vi "Weather Station UI.vi"(7 "stop":bool) -> (1 "Mise en garde":string, 2 "Historique de la température":dbl(graph))   [LabVIEW 2013]
doc: "Ceci est le VI principal du Projet Station météo. Il comporte l'interface utilisateur d'un système de mise en garde concernant la température. La température est mesurée toutes les demi-secondes ; les données sont enregistrées lorsqu'une mise en garde survient.\n\nEntrées utilisateur : Limite supérieure de température, Limite inférieure de température, Unités de température.\nSorties : Température actuelle, État de mise en garde."
uses:
  Supporting Files/Weather Station States.ctl
  Instance           1 26Saved   Weather Station UI .vi
panel:
  in  "Limite inférieure":dbl=10.0 min=0.0 max=50.0
  in  "Limite supérieure":dbl=30.0 min=0.0 max=50.0
  # "Gamme de température (C)"
  # "Canicule"
  # "Gel"
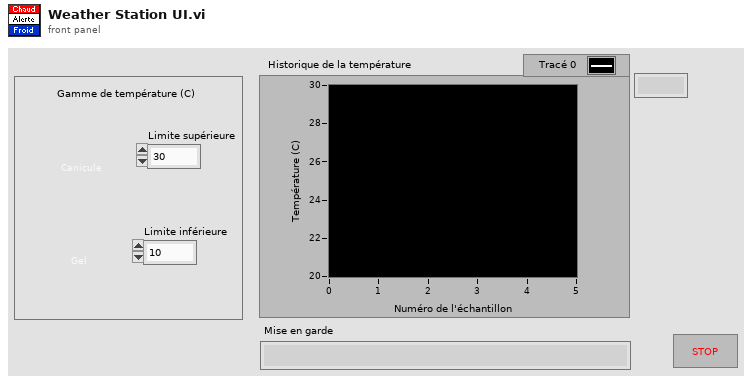
[diagram p1: front panel]
types:
  T1 = enum16{"open", "replace", "create", "open or create", "replace or create", "replace or create with confirmation"}
  T2 = typedef "Weather Station States.ctl" = enum16{"Acquisition", "Verification de la gamme", "Analyse", "Enregistrement des données", "Vérification du temps écoulé"}
  T3 = cluster{"Température":dbl, "Limite supérieure de T":dbl, "Limite inférieure de T":dbl, "Mise en garde":string}
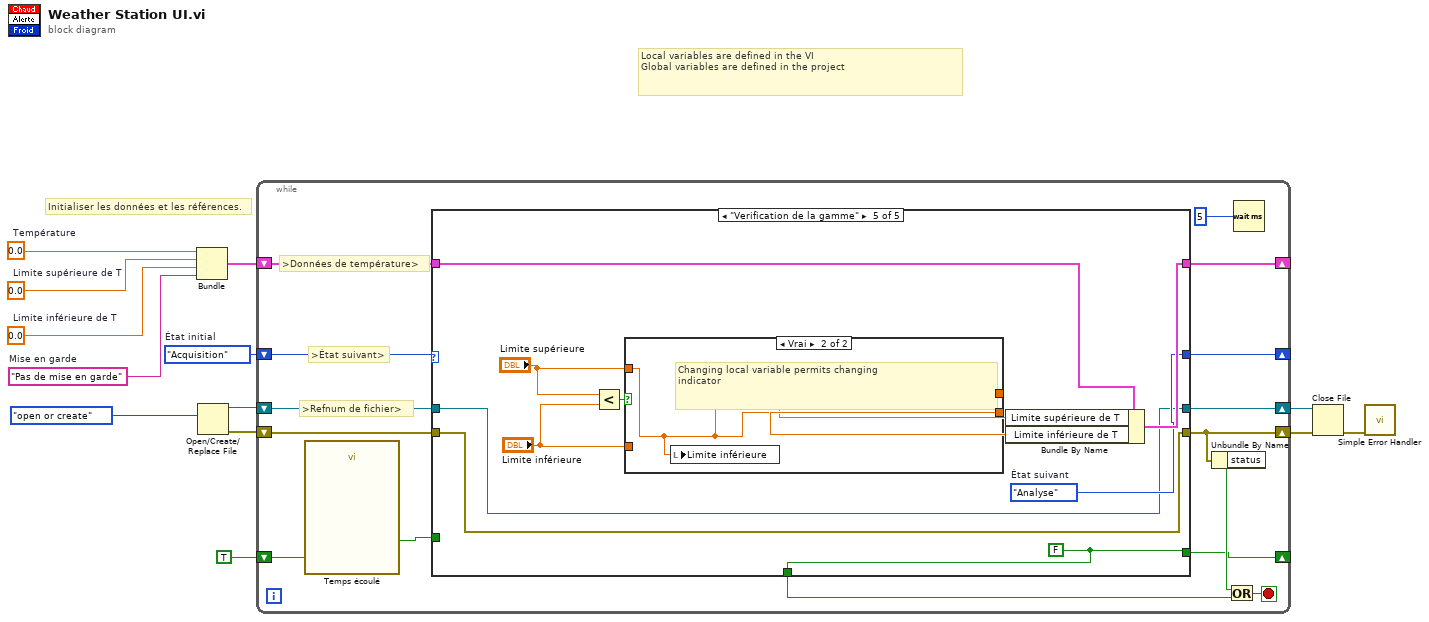
[diagram p0: block diagram]
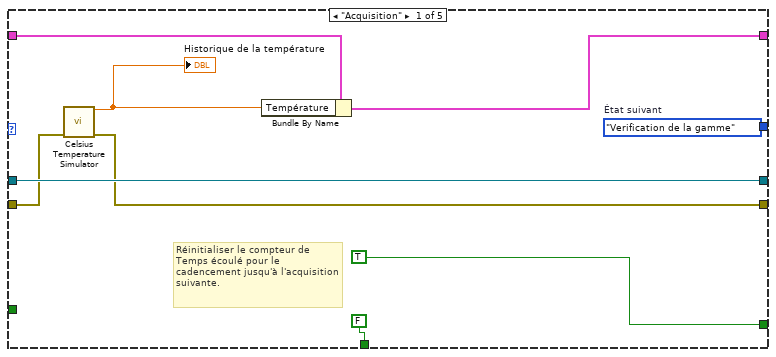
[diagram p2: hidden frame]
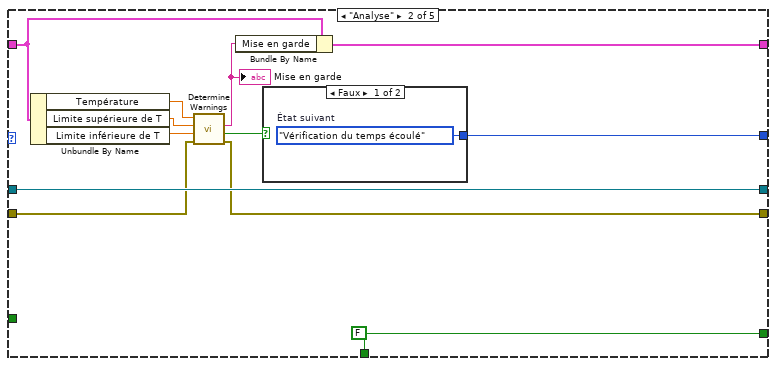
[diagram p3: hidden frame]
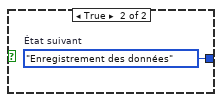
[diagram p4: hidden frame]
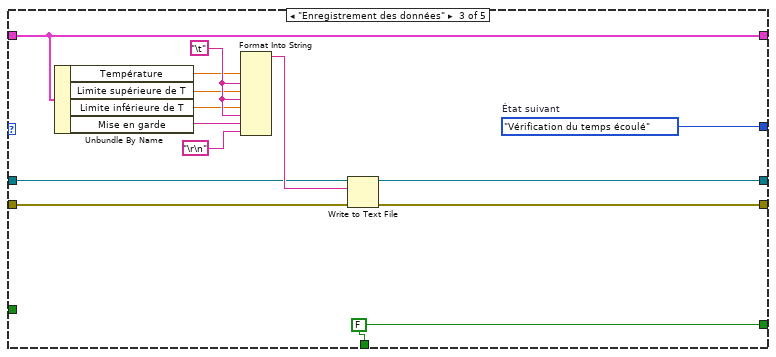
[diagram p5: hidden frame]
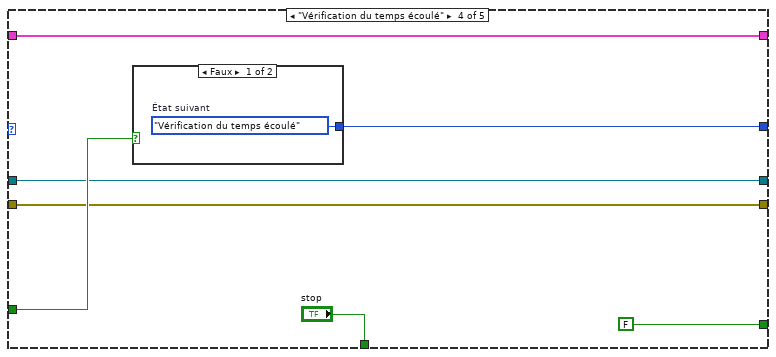
[diagram p6: hidden frame]
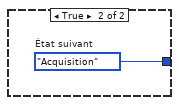
[diagram p7: hidden frame]
diagram:
  w7 = 0.0  # Limite inférieure de T
  w6 = 0.0  # Limite supérieure de T
  w8 = "Pas de mise en garde"  # Mise en garde
  w4 = 0.0  # Température
  w13 = Weather_Station_States."Acquisition"  # État initial
  # "Local variables are defined in the VI\nGlobal variables are defined in the project"
  # "Initialiser les données et les références."
  n1 = Bundle ("Assembler")("Température"=w4, "Limite supérieure de T"=w6, "Limite inférieure de T"=w7, "Mise en garde"=w8) -> (w1:T3)  [unwired: 1 out]
  n2 = Open/Create/Replace File ("Ouvrir/Créer/Remplacer un fichier")(operation (0:open)=T1."open or create") -> (refnum out=w3:refnum<file>, error out=w2:errorcluster)  [unwired: 1 in, 5 out]
  n3 = while "Boucle While" {
    shift-right: [w27] -> _
    shift-left: w13 -> [w28]
    shift-right: [w14] -> w12
    shift-left: w2 -> [w26]
    shift-right: [w15] -> _
    shift-left: w1 -> [w22]
    shift-right: [w23] -> w11
    shift-left: w3 -> [w21]
    shift-right: [w16] -> _
    shift-left: TRUE ("stop") -> [w18]
    stop <- w25 stop-if-true
    # ">Données de température>"
    # ">Refnum de fichier>"
    # ">État suivant>"
    n4 = call "Temps écoulé"("Reset"=w18) -> ("Time has Elapsed"=w17:bool)  [unwired: 4 in, 14 out]
    n5 = case "Structure Condition" shown="\"Verification de la gamme\"" w28 {
      tunnel: [w37 w47 w65 w71 w78] -> w27
      tunnel: [w29 w40 w63 w67 w77] -> w14
      tunnel: w26 -> [w30 w41 w64 w67 w77]
      tunnel: [w36 w49 w62 w68 w75] -> w23
      tunnel: [w32 w42 w52 w66 w79] -> w15
      tunnel: w22 -> [w33 w43 w52 w66 w82]
      tunnel: w21 -> [w36 w49 w60 w68 w75]
      tunnel: [FALSE ("stop") w48 w58 "stop" w76] -> w20
      tunnel: w17 -> [_ _ _ w72 _]
      tunnel: [TRUE ("stop") w48 w58 FALSE ("stop") w76] -> w16
      frame "Acquisition" {
        w37 = Weather_Station_States."Verification de la gamme"  # État suivant
        # "Réinitialiser le compteur de Temps écoulé pour le cadencement jusqu'à l'acquisition suivante."
        n6 = call "Celsius Temperature Simulator.vi"("entrée d'erreur (pas d'erreur)"=w30) -> ("Température"=w31:dbl, "sortie d'erreur"=w29:errorcluster)  [unwired: 13 out]
        "Historique de la température" <- w31
        n7 = Bundle By Name(cluster=w33, "Température"=w31) -> (w32:T3)
      }
      frame "Analyse" {
        w48 = FALSE ("stop")
        n8 = Unbundle By Name(w43) -> ("Température"=w46:dbl, "Limite supérieure de T"=w45:dbl, "Limite inférieure de T"=w44:dbl)
        n9 = call "Determine Warnings.vi"("entrée d'erreur (pas d'erreur)"=w41, "Temp. min."=w44, "Temp. max."=w45, "Temp. actuelle"=w46) -> ("sortie d'erreur"=w40:errorcluster, "Mise en garde ?"=w38:bool, "Texte de mise en garde"=w39:string)  [unwired: 5 out]
        "Mise en garde" <- w39
        n10 = Bundle By Name(cluster=w43, "Mise en garde"=w39) -> (w42:T3)
        n11 = case shown="Faux" w38 {
          tunnel: [w50 w51] -> w47
          frame False {
            w50 = Weather_Station_States."Vérification du temps écoulé"  # État suivant
          }
          frame True {
            w51 = Weather_Station_States."Enregistrement des données"  # État suivant
          }
        }
      }
      frame "Enregistrement des données" {
        w65 = Weather_Station_States."Vérification du temps écoulé"  # État suivant
        w58 = FALSE ("stop")
        w59 = "\t"
        n12 = Unbundle By Name(w52) -> ("Température"=w57:dbl, "Limite supérieure de T"=w56:dbl, "Limite inférieure de T"=w55:dbl, "Mise en garde"=w54:string)
        n13 = Format Into String(w57, w59, w56, w59, w55, w59, w54, "\r\n") -> (resulting string=w61:string)  [unwired: 3 in, 1 out]
        n14 = Write to Text File(file (use dialog)=w60, text=w61, error in=w64) -> (refnum out=w62:refnum<file>, error out=w63:errorcluster)  [unwired: 2 out]
      }
      frame "Vérification du temps écoulé" {
        n15 = case shown="Faux" w72 {
          tunnel: [w73 w74] -> w71
          frame False {
            w73 = Weather_Station_States."Vérification du temps écoulé"  # État suivant
          }
          frame True {
            w74 = Weather_Station_States."Acquisition"  # État suivant
          }
        }
      }
      frame "Verification de la gamme" {
        w76 = FALSE
        w78 = Weather_Station_States."Analyse"  # État suivant
        n16 = Less?(x="Limite supérieure", y="Limite inférieure") -> (x < y?=w85:bool)
        n17 = case shown="Vrai" w85 {
          tunnel: "Limite inférieure" -> [w86 _]
          tunnel: "Limite supérieure" -> [w87 w88]
          tunnel: [w86 w88] -> w81
          tunnel: [w87 w88] -> w80
          frame False {
          }
          frame True {
            # "Changing local variable permits changing\nindicator"
            n18 = local write "Limite inférieure"(w88) -> ()
          }
        }
        n19 = Bundle By Name(cluster=w82, "Limite supérieure de T"=w80, "Limite inférieure de T"=w81) -> (w79:T3)
      }
    }
    n20 = Unbundle By Name ("Désassembler par nom")(w14) -> ("status"=w24:bool)
    n21 = Or ("OU")(x=w24, y=w20) -> (x .or. y?=w25:bool)
    n22 = Wait (ms) ("Attendre (ms)")(milliseconds to wait=u32 5 ("y")) -> ()  [unwired: 1 out]
  }
  n23 = Close File ("Fermer un fichier")(refnum=w11, error in=w12) -> (error out=w10:errorcluster)  [unwired: 1 out]
  n24 = call <vilib>:"Simple Error Handler.vi"("error in (no error)"=w10) -> ()  [unwired: 1 in, 8 out]
